vi "primer_programa.vi"() -> ()   [LabVIEW 2013]
panel:
  out "Waveform Chart":dbl(graph)
  out "Gauge":dbl(knob) scale=0.0..500.0
  out "Tank":dbl(slide) scale=0.0..500.0
  in  "ingresar datos":dbl(knob) caption="Knob" scale=0.0..500.0
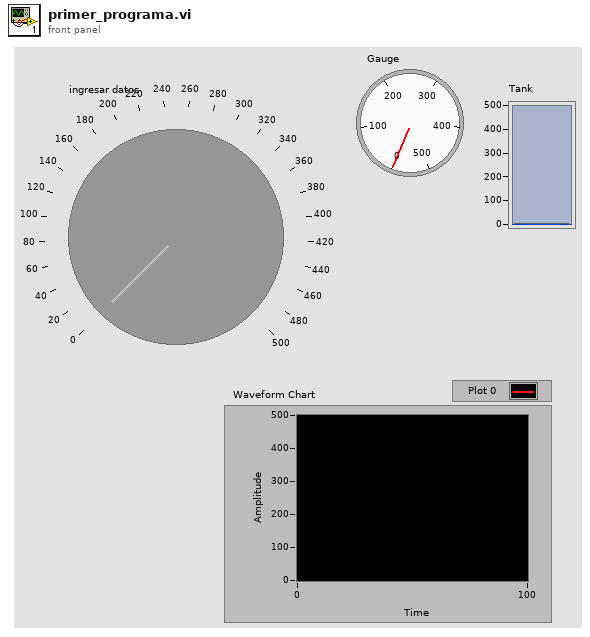
[diagram p1: front panel]
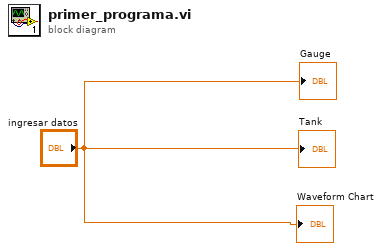
[diagram p0: block diagram]
diagram:
  "Tank" <- "ingresar datos"
  "Gauge" <- "ingresar datos"
  "Waveform Chart" <- "ingresar datos"
